vi "tank.vi"() -> ()   [LabVIEW 2018]
uses:
  <vilib>/addons/Fuzzy Logic/FL Fuzzy Controller (MISO).vi
  <vilib>/addons/Fuzzy Logic/NI_Fuzzy_Logic_API.lvlib
panel:
  in  "Tank Set Point":dbl(slide) scale=0.0..5.0 scale format="%#_2g"
  out "rule weights":dbl[](array[numeric])
  in  "Stop":bool
  out "Simulated dT(s)":dbl=0.021
  out "Tank":dbl(slide)=0.4094942850910191 scale=0.0..5.0 scale format="%#.1f"
  out "Flow Rate":dbl(knob)=0.3538687715086328 min=0.0 max=0.5 step=0.05 scale=0.0..5.0 scale format="%#.1f"
  out "Process Monitor":T1(graph)
  out "Valve":bool
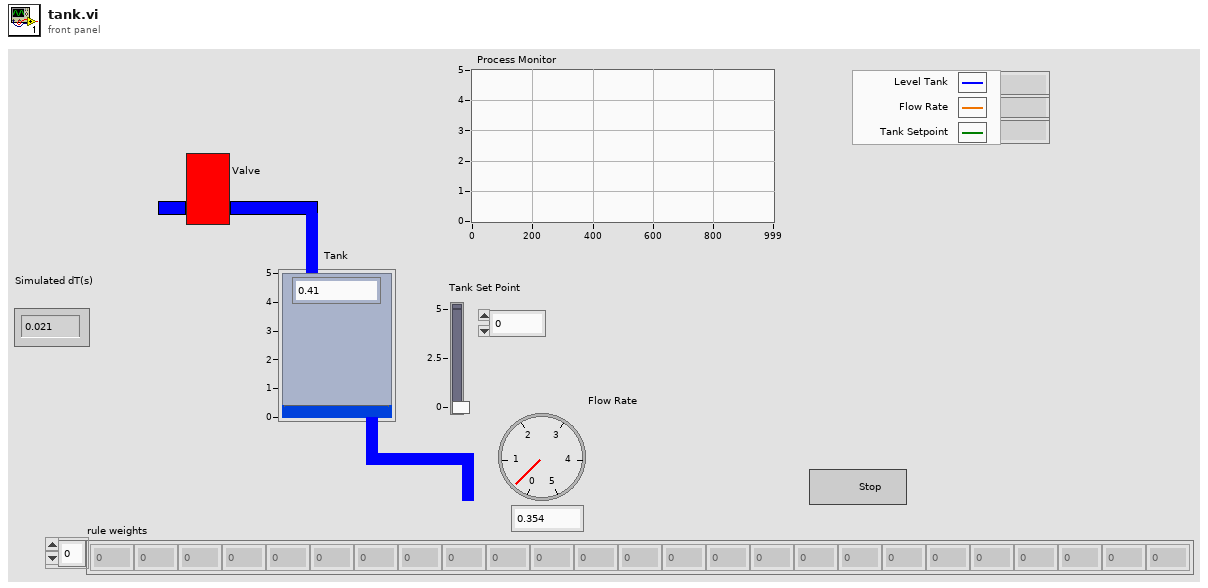
[diagram p1: front panel]
types:
  T1 = cluster{"hnew":dbl, "Flow Rate In":dbl, "Tank 2 Set Point":dbl}
  T2 = typedef "NI_Fuzzy_Logic_API.lvlib/FL System.ctl" = cluster{"input variables":T3[], "output variables":T3[], "rules":T6[], "defuzzification method":T12, "description":string, "user MF interpolating polynomials":T13[]}
  T3 = typedef "NI_Fuzzy_Logic_API.lvlib/FL Variable.ctl" = cluster{"name":string, "range":dbl[], "MFs":T4[]}
  T4 = typedef "NI_Fuzzy_Logic_API.lvlib/FL Membership Function.ctl" = cluster{"name":string, "shape":T5, "points":dbl[], "color":u32, "user-defined shape index":i32}
  T5 = typedef "NI_Fuzzy_Logic_API.lvlib/FL Membership Function Shape.ctl" = u16
  T6 = typedef "NI_Fuzzy_Logic_API.lvlib/FL Rule.ctl" = cluster{"antecedents":T7[], "antecedent connective":T9, "consequents":T10[], "consequent implication":T11, "degree of support":dbl}
  T7 = typedef "NI_Fuzzy_Logic_API.lvlib/FL Antecedent.ctl" = cluster{"Var Index":i32, "MF Index":i32, "Cond":T8}
  T8 = typedef "NI_Fuzzy_Logic_API.lvlib/FL Modifier.ctl" = u16
  T9 = typedef "NI_Fuzzy_Logic_API.lvlib/FL Antecedent Connective.ctl" = u16
  T10 = typedef "NI_Fuzzy_Logic_API.lvlib/FL Consequent.ctl" = cluster{"Var Index":i32, "MF Index":i32, "Cond":T8}
  T11 = typedef "NI_Fuzzy_Logic_API.lvlib/FL Consequent Implication.ctl" = u16
  T12 = typedef "NI_Fuzzy_Logic_API.lvlib/FL Defuzzification.ctl" = u16
  T13 = typedef "NI_Fuzzy_Logic_API.lvlib/FL Interpolating polynomials.ctl" = cluster{"X":dbl[], "Y":dbl[], "Y(x) coeff":dbl[][], "X(y) coeff":dbl[][], "Area(y) coeff":dbl[][], "coa_x(y) coeff":dbl[][]}
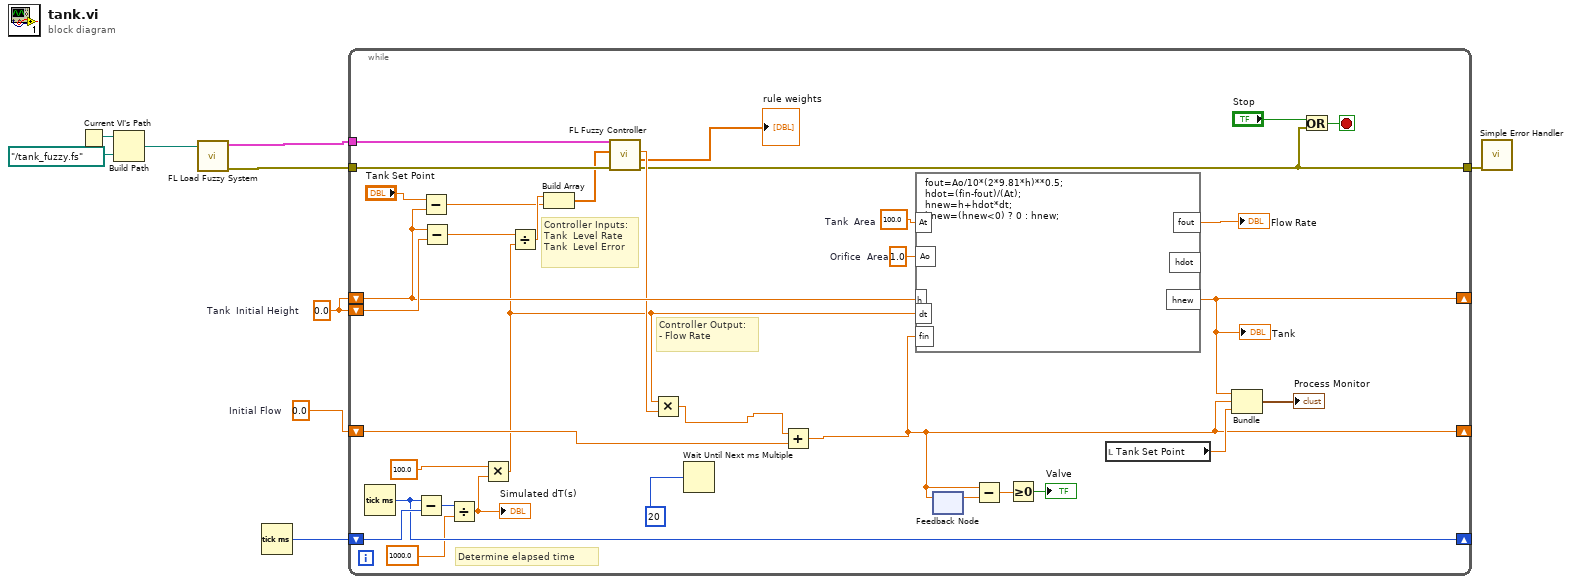
[diagram p0: block diagram]
diagram:
  w6 = 0.0  # Initial Flow
  w8 = 0.0  # Tank  Initial Height
  n1 = Current VI's Path() -> (path=w4:path)
  n2 = Build Path(base path=w4, name or relative path=path "../tank_fuzzy.fs") -> (appended path=w3:path)
  n3 = call <vilib>:"FL Load Fuzzy System.vi"("file path"=w3) -> ("error out"=w1:errorcluster, "fuzzy system out"=w2:T2)  [unwired: 1 in, 8 out]
  n4 = Tick Count (ms)() -> (millisecond timer value=w9:u32)
  n5 = while {
    shift-left: w8 -> [w39]
    shift-left: w6 -> [w40]
    shift-right: [w13] -> _
    tunnel: w2 -> [w41]
    shift-left: w9 -> [w43]
    shift-right: [w38] -> _
    shift-left: w8 -> [w37]
    shift-right: [w42] -> _
    tunnel: w1 -> [w27]
    tunnel: [w16] -> w7
    stop <- w17 stop-if-true
    w31 = 1.0  # Orifice  Area
    w32 = 100.0  # Tank  Area
    # "Controller Inputs:\nTank  Level Rate\nTank  Level Error"
    # "Controller Output:\n- Flow Rate"
    # "Determine elapsed time"
    n6 = Tick Count (ms)() -> (millisecond timer value=w38:u32)
    n7 = Subtract(x=w38, y=w43) -> (x-y=w28:u32)
    n8 = Subtract(x="Tank Set Point", y=w37) -> (x-y=w23:dbl)
    n9 = Subtract(x=w37, y=w39) -> (x-y=w33:dbl)
    n10 = Divide(x=w28, y=1000.0) -> (x/y=w35:dbl)
    "Simulated dT(s)" <- w35
    n11 = Multiply(x=100.0, y=w35) -> (x*y=w22:dbl)
    n12 = Divide(x=w33, y=w22) -> (x/y=w24:dbl)
    n13 = Build Array(w24, w23) -> (w26:dbl[])
    n14 = call-poly <vilib>:"FL Fuzzy Controller.vi"("error in (no error)"=w27, "input values"=w26, "fuzzy system in"=w41) -> ("error out"=w16:errorcluster, "rule weights"=→"rule weights":dbl[], "output value"=w25:dbl)  [unwired: 6 out]
    n15 = Multiply(x=w22, y=w25) -> (x*y=w12:dbl)
    n16 = Wait Until Next ms Multiple(millisecond multiple=u32 20) -> ()  [unwired: 1 out]
    n17 = Add(x=w12, y=w40) -> (x+y=w13:dbl)
    n18 = formula code="fout=Ao/10*(2*9.81*h)**0.5;\nhdot=(fin-fout)/(At);\nhnew=h+hdot*dt;\nhnew=(hnew<0) ? 0 : hnew;"("fin"=w13, "h"=w37, "At"=w32, "Ao"=w31, "dt"=w22) -> ("fout"=→"Flow Rate":dbl, "hnew"=w42:dbl)  [unwired: 1 out]
    "Tank" <- w42
    n19 = feedback-in #1(w13) -> ()
    n20 = feedback #1() -> (w21:dbl)  [unwired: 1 in]
    n21 = Subtract(x=w13, y=w21) -> (x-y=w20:dbl)
    n22 = Greater Or Equal To 0?(x=w20) -> (x >= 0?=→"Valve":bool)
    n23 = local read "Tank Set Point"() -> (w29:dbl)
    n24 = Bundle("hnew"=w42, w13, "Tank Set Point"=w29) -> (→"Process Monitor":cluster{"hnew":dbl, dbl, "Tank Set Point":dbl})  [unwired: 1 out]
    n25 = Or(x="Stop", y=w16) -> (x .or. y?=w17:bool)
  }
  n26 = call <vilib>:"Simple Error Handler.vi"("error in (no error)"=w7) -> ()  [unwired: 4 in, 5 out]
